vi "Write fixed timing source name.vi"(8 "error in":errorcluster, 10 "fixed timing source name":string, 11 "DecideProjectFeatures in":refnum<class "UserTBModuleDecideFeatures.lvclass">) -> (0 "error out":errorcluster, 3 "DecideProjectFeatures out":refnum<class "UserTBModuleDecideFeatures.lvclass">)   [LabVIEW 2013, in "UserTBModuleDecideFeatures.lvclass"]
uses:
  UserTBModuleDecideFeatures.lvclass
  UserTBModuleDecideFeatures.lvclass/UserTBModuleDecideFeatures.ctl
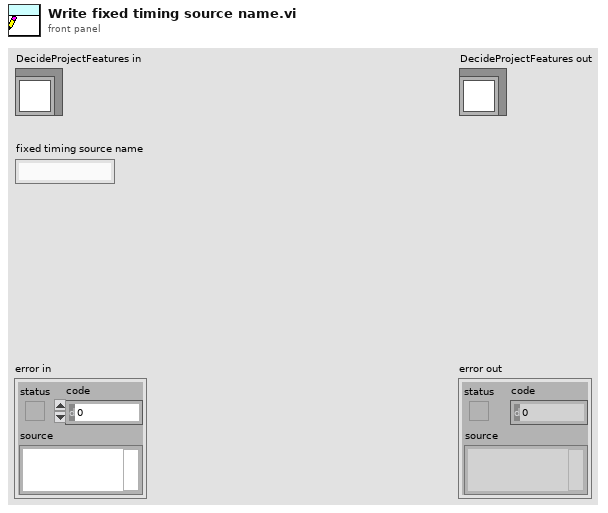
[diagram p1: front panel]
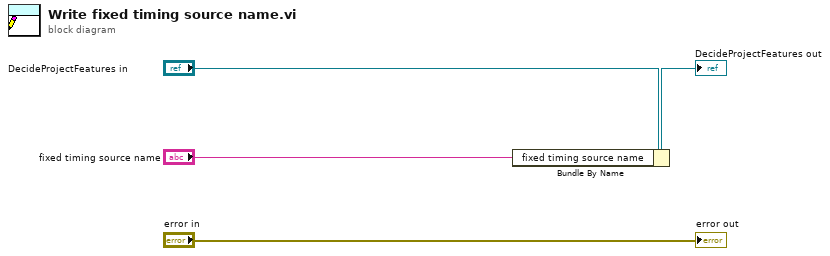
[diagram p0: block diagram]
diagram:
  n1 = Bundle By Name(cluster="DecideProjectFeatures in", "fixed timing source name"="fixed timing source name") -> (→"DecideProjectFeatures out":refnum<class "UserTBModuleDecideFeatures.lvclass">)
  "error out" <- "error in"
